vi "Scan DNS Config.vi"(8 "error in (no error)":errorcluster) -> (0 "error out":errorcluster, 3 "DNS server addresses":refnum<class "Generic Network Address.lvclass">[](array[class]), 4 "found?":bool)   [LabVIEW 2020, in "NI_WFCN.lvlib" / "Hostname Network Address.lvclass"]
doc: "Search for configured DNS servers."
uses:
  <vilib>/net/WFCN/Addressing/Hostname Network Address/Hostname Network Address.lvclass
  <vilib>/net/WFCN/Addressing/Generic Network Address/Generic Network Address.lvclass
  <vilib>/net/WFCN/Addressing/Hostname Network Address/Windows run ipconfig.vi
  <vilib>/net/WFCN/Addressing/Hostname Network Address/Parse ipconfig.vi
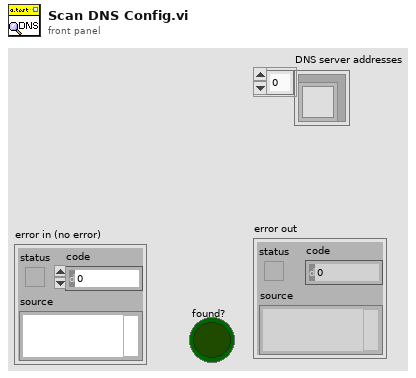
[diagram p1: front panel]
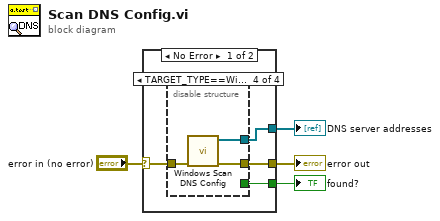
[diagram p0: block diagram]
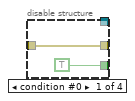
[diagram p2: hidden frame]
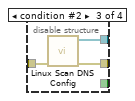
[diagram p4: hidden frame]
diagram:
  n1 = case shown="No Error" "error in (no error)" {
    selector: "error in (no error)" -> [w8 w18]
    tunnel: [w7 w18] -> w3
    tunnel: [w5 _] -> w2
    tunnel: [w6 _] -> w1
    frame No Error {
      n2 = disable-structure "Conditional Disable Structure" shown="TARGET_TYPE==Windows" {
        disable-tunnel: w8 -> [w10 w11 w14 w17]
        disable-tunnel: [w10 w11 w13 w15] -> w7
        disable-tunnel: [_ _ w12 w16] -> w5
        disable-tunnel: [TRUE _ _ _] -> w6
        frame condition #0 {
        }
        frame condition #1 {
        }
        frame condition #2 {
          n3 = call <vilib>:"Linux Scan DNS Config.vi"("error in (no error)"=w14) -> ("error out"=w13:errorcluster, "DNS server addresses"=w12:refnum<class "Generic Network Address.lvclass">[])  [unwired: 9 in]
        }
        frame condition #3 (active) {
          n4 = call <vilib>:"Windows Scan DNS Config.vi"("error in (no error)"=w17) -> ("error out"=w15:errorcluster, "DNS server addresses"=w16:refnum<class "Generic Network Address.lvclass">[])  [unwired: 9 in]
        }
      }
    }
    frame Error {
    }
  }
  "error out" <- w3
  "DNS server addresses" <- w2
  "found?" <- w1
